vi "Handle Debug Data.vi"(8 "error in (no error)":errorcluster, 10 "Debug Data.lvclass":refnum<class "Debug Data.lvclass">, 11 "Debug Data Event In":refnum<class "Debug Data Listener.lvclass">) -> (0 "error out":errorcluster, 3 "Debug Data Event Out":refnum<class "Debug Data Listener.lvclass">)   [LabVIEW 2020, in "Debug Data Listener.lvclass"]
uses:
  Debug Data Listener.lvclass
  Debug Data/Debug Data.lvclass
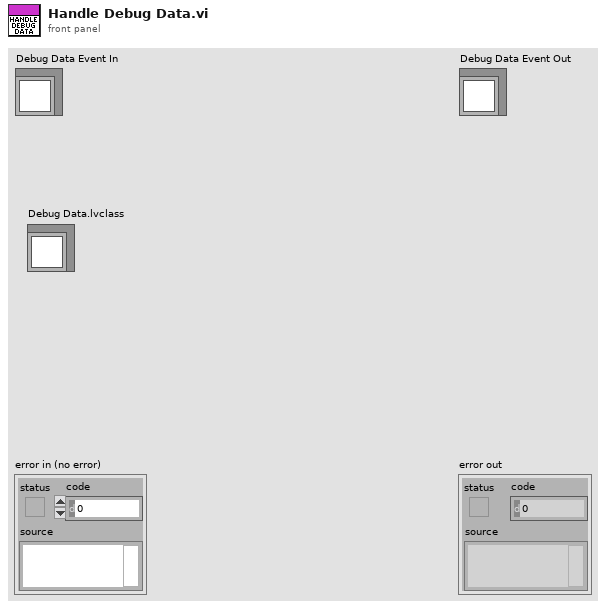
[diagram p1: front panel]
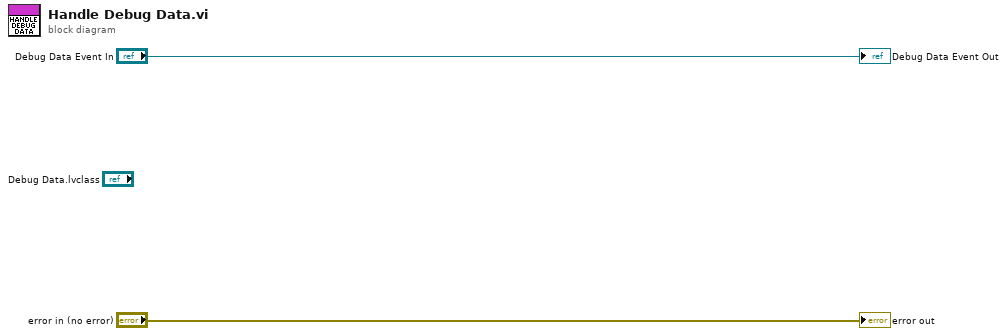
[diagram p0: block diagram]
diagram:
  "error out" <- "error in (no error)"
  "Debug Data Event Out" <- "Debug Data Event In"
